vi "tcpip_forward.vi"() -> ()   [LabVIEW 2013]
uses:
  libssh2/libssh2.lvlib
panel:
  in  "stop":bool
  in  "local_destport":i32=4444
  in  "local_destip":string="localhost"
  in  "remote_wantport":i32=2222
  in  "remote_listenhost":string="localhost"
  in  "server_ip":string="127.0.0.1"
  in  "password":string
  in  "username":string
  out "error out":errorcluster
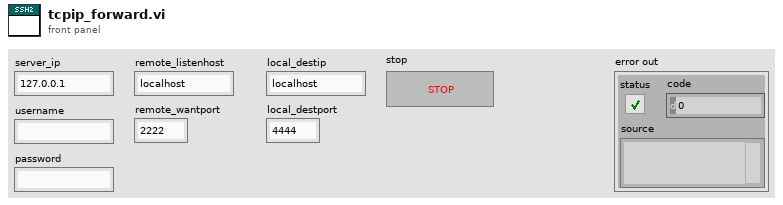
[diagram p1: front panel]
types:
  T1 = typedef "libssh2.lvlib/Session Refnum.ctl" = refnum<k1>
  T2 = typedef "libssh2.lvlib/Listener Refnum.ctl" = refnum<k1>
  T3 = typedef "libssh2.lvlib/Channel Refnum.ctl" = refnum<k1>
  T4 = enum16{"Standard", "Buffered", "CRLF", "Immediate"}
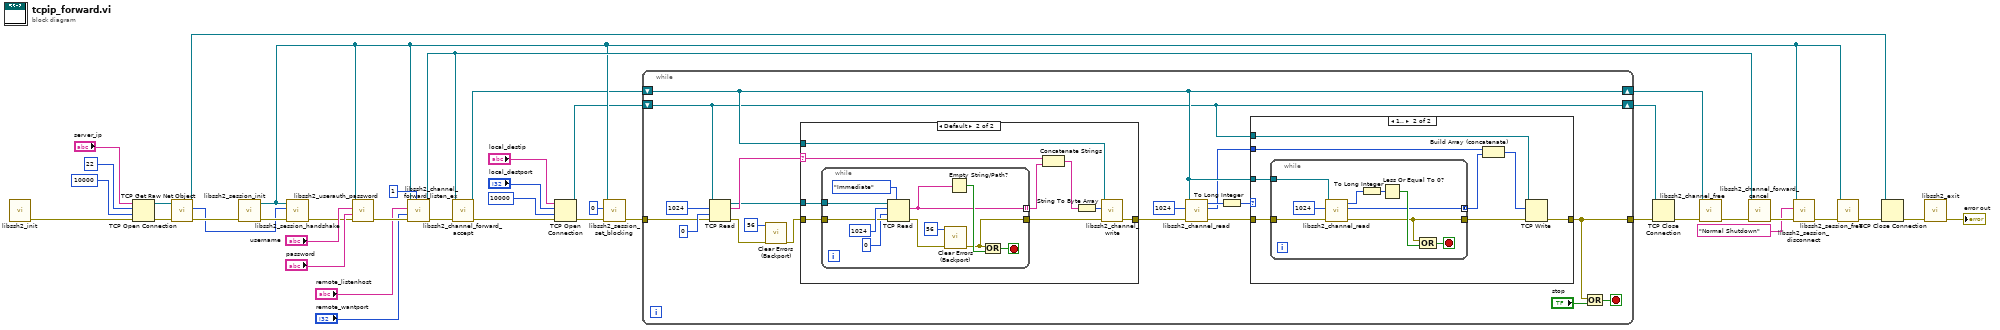
[diagram p0: block diagram]
diagram:
  n1 = call "libssh2_init.vi"() -> ("error out"=w35:errorcluster)  [unwired: 10 in, 1 out]
  n2 = TCP Open Connection(address="server_ip", remote port or service name=u16 22, timeout ms (60000)=10000, error in (no error)=w35) -> (connection ID=w37:refnum<k5>, error out=w36:errorcluster)  [unwired: 1 in]
  n3 = call <vilib>:"TCP Get Raw Net Object.vi"("error in (no error)"=w36, "connection ID"=w37) -> ("error out"=w34:errorcluster, "raw net object"=w32:u64, "connection ID out"=w30:refnum<k5>)  [unwired: 7 in]
  n4 = call "libssh2_session_init.vi"("error in (no error)"=w34) -> ("error out"=w33:errorcluster, "session"=w6:T1)  [unwired: 9 in]
  n5 = call "libssh2_session_handshake.vi"("error in (no error)"=w33, "socket"=w32, "session"=w6) -> ("error out"=w10:errorcluster)  [unwired: 7 in, 1 out]
  n6 = call "libssh2_userauth_password.vi"("error in (no error)"=w10, "password"="password", "username"="username", "session"=w6) -> ("error out"=w29:errorcluster)  [unwired: 6 in, 1 out]
  n7 = call "libssh2_channel_forward_listen_ex.vi"("queue_maxsize"=1, "error in (no error)"=w29, "port"="remote_wantport", "host"="remote_listenhost", "session"=w6) -> ("error out"=w25:errorcluster, "listener"=w20:T2)  [unwired: 4 in, 1 out]
  n8 = call "libssh2_channel_forward_accept.vi"("error in (no error)"=w25, "listener"=w20) -> ("error out"=w24:errorcluster, "channel"=w3:T3)  [unwired: 8 in]
  n9 = TCP Open Connection(address="local_destip", remote port or service name="local_destport", timeout ms (60000)=10000, error in (no error)=w24) -> (connection ID=w2:refnum<k5>, error out=w8:errorcluster)  [unwired: 1 in]
  n10 = call "libssh2_session_set_blocking.vi"("error in (no error)"=w8, "blocking"=0, "session"=w6) -> ("error out"=w7:errorcluster)  [unwired: 8 in]
  n11 = while {
    tunnel: w7 -> [w48]
    tunnel: [w43] -> w1
    shift-right: [w51] -> w5
    shift-left: w3 -> [w51]
    shift-right: [w45] -> w4
    shift-left: w2 -> [w45]
    stop <- w41 stop-if-true
    n12 = TCP Read(connection ID=w45, bytes to read=1024, error in (no error)=w48, 9:0 ("timeout ms (25000)")) -> (connection ID out=w46:refnum<k5>, data out=w58:string, error out=w50:errorcluster)  [unwired: 1 in]
    n13 = call "Clear Errors (Backport).vi"("error in (no error)"=w50, "specific error code to clear (0: all)"=56) -> ("error out"=w47:errorcluster)  [unwired: 4 in, 1 out]
    n14 = case shown="Default" w58 {
      selector: w58 -> [_ w81]
      tunnel: [w78 w84] -> w54
      tunnel: w46 -> [_ w87]
      tunnel: w47 -> [w78 w86]
      tunnel: w51 -> [_ w83]
      frame "" {
      }
      frame Default {
        n15 = while {
          tunnel: [w89] -> w85
          tunnel: w87 -> [w96]
          tunnel: w86 -> [w93]
          tunnel: [w88] -> w82 mode=indexing
          stop <- w94 stop-if-true
          n16 = TCP Read(connection ID=w96, bytes to read=1024, error in (no error)=w93, 7:T4."Immediate" ("mode (standard)"), 9:0 ("timeout ms (25000)")) -> (data out=w88:string, error out=w90:errorcluster)  [unwired: 1 out]
          n17 = call "Clear Errors (Backport).vi"("error in (no error)"=w90, "specific error code to clear (0: all)"=56) -> ("error out"=w89:errorcluster)  [unwired: 4 in, 1 out]
          n18 = Empty String/Path?(string/path=w88) -> (empty?=w95:bool)
          n19 = Or(x=w89, y=w95) -> (x .or. y?=w94:bool)
        }
        n20 = Concatenate Strings(w81, w82) -> (w80:string)
        n21 = String To Byte Array(string=w80) -> (unsigned byte array=w79:u8[])
        n22 = call "libssh2_channel_write.vi"("error in (no error)"=w85, "buf"=w79, "channel"=w83) -> ("error out"=w84:errorcluster)  [unwired: 7 in, 1 out]
      }
    }
    n23 = call "libssh2_channel_read.vi"("error in (no error)"=w54, "buflen"=u64 1024, "channel"=w51) -> ("error out"=w53:errorcluster, "buf"=w44:u8[], "return value"=w52:i64)  [unwired: 6 in]
    n24 = To Long Integer(number=w52) -> (32bit integer=w56:i32)
    n25 = case shown="1.." w56 {
      tunnel: [w60 w66] -> w43
      tunnel: w51 -> [_ w68]
      tunnel: w45 -> [_ w65]
      tunnel: w53 -> [w60 w67]
      tunnel: w44 -> [_ w64]
      frame Default {
      }
      frame 1.. {
        n26 = while {
          tunnel: w68 -> [w72]
          tunnel: w67 -> [w73]
          tunnel: [w70] -> w63 mode=concatenating
          tunnel: [w69] -> w61
          stop <- w77 stop-if-true
          n27 = call "libssh2_channel_read.vi"("error in (no error)"=w73, "buflen"=u64 1024, "channel"=w72) -> ("error out"=w69:errorcluster, "buf"=w70:u8[], "return value"=w71:i64)  [unwired: 6 in]
          n28 = To Long Integer(number=w71) -> (32bit integer=w75:i32)
          n29 = Less Or Equal To 0?(x=w75) -> (x <= 0?=w76:bool)
          n30 = Compound Arithmetic op=OR(w69, w76) -> (w77:bool)
        }
        n31 = Build Array (concatenate)(w64, w63) -> (w62:u8[])
        n32 = TCP Write(connection ID=w65, data in=w62, error in (no error)=w61) -> (error out=w66:errorcluster)  [unwired: 1 in, 2 out]
      }
    }
    n33 = Or(x=w43, y="stop") -> (x .or. y?=w41:bool)
  }
  n34 = TCP Close Connection(connection ID=w4, error in (no error)=w1) -> (error out=w18:errorcluster)  [unwired: 1 in, 1 out]
  n35 = call "libssh2_channel_free.vi"("error in (no error)"=w18, "channel"=w5) -> ("error out"=w21:errorcluster)  [unwired: 8 in, 1 out]
  n36 = call "libssh2_channel_forward_cancel.vi"("error in (no error)"=w21, "listener"=w20) -> ("error out"=w19:errorcluster)  [unwired: 8 in, 1 out]
  n37 = call "libssh2_session_disconnect.vi"("error in (no error)"=w19, "description"="Normal Shutdown", "session"=w6) -> ("error out"=w31:errorcluster)  [unwired: 7 in, 1 out]
  n38 = call "libssh2_session_free.vi"("error in (no error)"=w31, "session"=w6) -> ("error out"=w11:errorcluster)  [unwired: 8 in, 1 out]
  n39 = TCP Close Connection(connection ID=w30, error in (no error)=w11) -> (error out=w13:errorcluster)  [unwired: 1 in, 1 out]
  n40 = call "libssh2_exit.vi"("error in (no error)"=w13) -> ("error out"=→"error out":errorcluster)  [unwired: 10 in]
